vi "GenerateCode.vi"() -> ()   [LabVIEW 2018]
panel:
  in  "RegenerateAll":bool
  # "Select RegenerateAll to regenerate all of your CommandTemplates.\nIf RegenerateAll is false, the program will try to use Git and a file\nnamed LastGeneratedDates.ini to figure out which files should be \nregenerated because changes were made to them. This feature is enabled\nby default inside of GenerateCommandsFromTemplates.vi. If you do not have\nGit please disable this feature. The code will then always RegenerateAll."
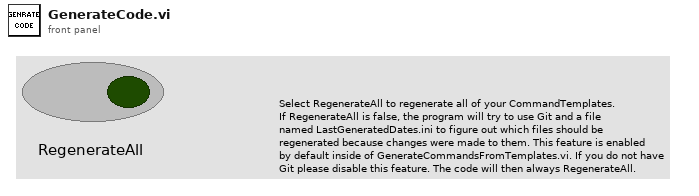
[diagram p1: front panel]
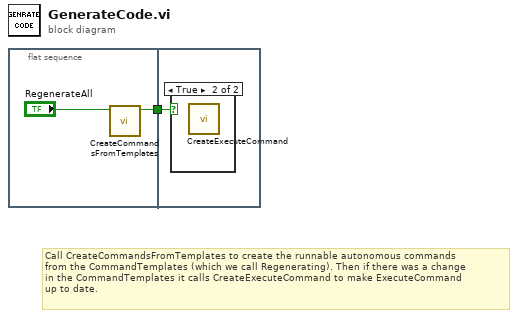
[diagram p0: block diagram]
diagram:
  # "Call CreateCommandsFromTemplates to create the runnable autonomous commands\nfrom the CommandTemplates (which we call Regenerating). Then if there was a change\nin the CommandTemplates it calls CreateExecuteCommand to make ExecuteCommand\nup to date."
  n1 = flat-sequence {
    tunnel: [w3] -> w1
    tunnel: w1 -> [w4]
    frame #0 {
      n2 = call "CreateCommandsFromTemplates.vi"("RegenerateAll"="RegenerateAll") -> ("NewVI"=w3:bool)  [unwired: 10 in]
    }
    frame #1 {
      n3 = case shown="True" w4 {
        frame False {
        }
        frame True {
          n4 = call "CreateExecuteCommand.vi"() -> ()  [unwired: 12 in]
        }
      }
    }
  }
